vi "Configure Rotate Bits.vi"(6 "Enable Waveform (T: Enable)":bool=TRUE, 7 "Walk Value (0: Zeroes)":i32(ring) items=["Zeroes", "Ones"], 8 "error in (no error)":errorcluster, 9 "Dwell (1)":i32=1, 10 "Channel (0: chA)":i32(ring) items=["chA", "chB"], 11 "VISA resource name":refnum<visa-resource-name>) -> (0 "error out":errorcluster, 3 "VISA resource name out":refnum<visa-resource-name>)   [LabVIEW 2014, in "Stanford Research SR1.lvlib"]
doc: "Configures the attributes for the Rotate Bits."
uses:
  Stanford Research SR1.lvlib
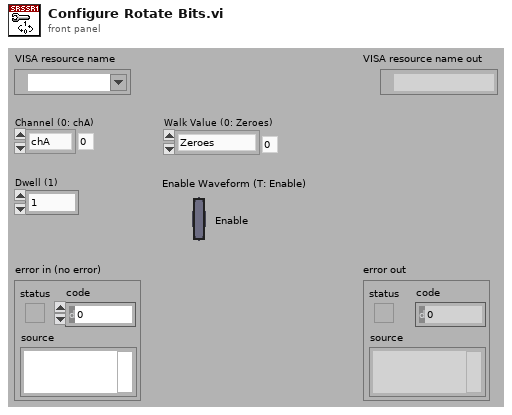
[diagram p1: front panel]
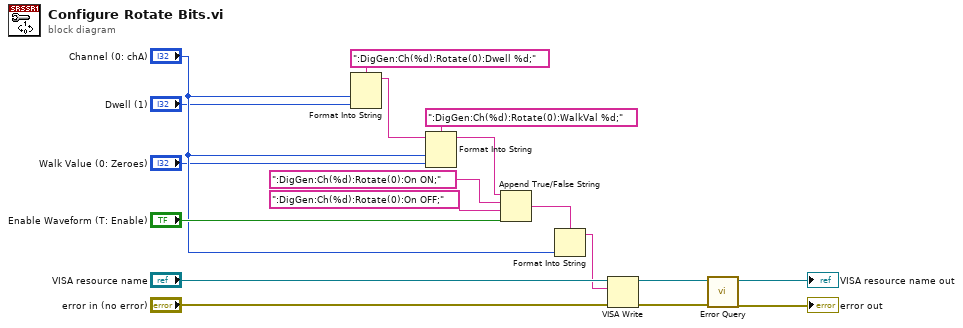
[diagram p0: block diagram]
diagram:
  n1 = Format Into String(format string=":DigGen:Ch(%d):Rotate(0):Dwell %d;", "Channel (0: chA)", "Dwell (1)") -> (resulting string=w17:string)  [unwired: 2 in, 1 out]
  n2 = Format Into String(format string=":DigGen:Ch(%d):Rotate(0):WalkVal %d;", initial string=w17, "Channel (0: chA)", "Walk Value (0: Zeroes)") -> (resulting string=w15:string)  [unwired: 1 in, 1 out]
  n3 = Append True/False String(1:"Enable Waveform (T: Enable)", 2:":DigGen:Ch(%d):Rotate(0):On OFF;", 3:":DigGen:Ch(%d):Rotate(0):On ON;", 4:w15) -> (0:w5:string)
  n4 = Format Into String(format string=w5, "Channel (0: chA)") -> (resulting string=w4:string)  [unwired: 2 in, 1 out]
  n5 = VISA Write(VISA resource name="VISA resource name", write buffer=w4, error in (no error)="error in (no error)") -> (VISA resource name out=w9:refnum<visa-resource-name>, error out=w8:errorcluster)  [unwired: 1 out]
  n6 = call "Error Query.vi"("error in (no error)"=w8, "VISA resource name"=w9) -> ("error out"=→"error out":errorcluster, "VISA resource name out"=→"VISA resource name out":refnum<visa-resource-name>)  [unwired: 6 in, 2 out]
